vi "Write Scan Configuration.vi"(8 "error in (no error)":errorcluster, 10 "Configuration":T1={"Start"=-0.001, "End"=0.001, "Step"=0.0001, "Delta"=0.0001, "Scan shape"=enum."Sawtooth", "Append measurements"=[]} {"Delta" format="%#_6p"; "Step" format="%#_6p"; "End" format="%#_6p"; "Start" format="%#_6p"}, 11 "Keithley 622x2182 Driver in":refnum<class "Keithley 622x2182 Driver.lvclass">) -> (0 "error out":errorcluster, 3 "Keithley 622x2182 Driver out":refnum<class "Keithley 622x2182 Driver.lvclass">)   [LabVIEW 2021, in "Keithley 622x2182 Driver.lvclass"]
uses:
  Keithley 622x2182 Driver.lvclass
  C:/Git/NHMFL_Core/Libraries/Instruments/Instrument Driver/Instrument Driver.lvclass
  Controls/Stepper Config.ctl
  Keithley 622x2182 Driver.lvclass/Keithley 622x2182 Driver.ctl
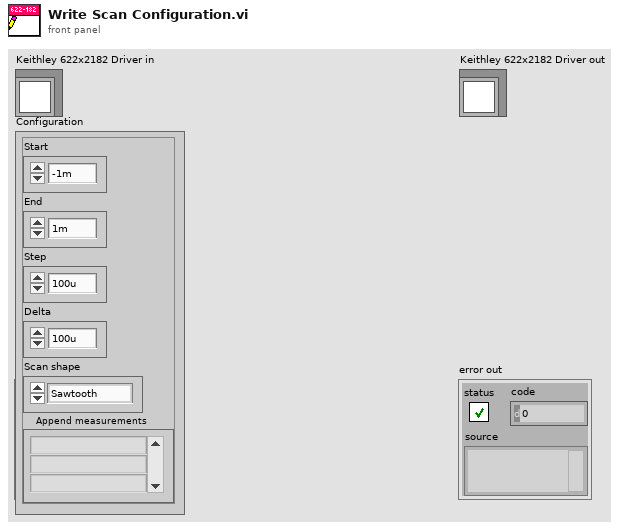
[diagram p1: front panel]
types:
  T1 = typedef "Stepper Config.ctl" = cluster{"Start":dbl, "End":dbl, "Step":dbl, "Delta":dbl, "Scan shape":enum16{"Sawtooth", "Triangular"}, "Append measurements":string[]}
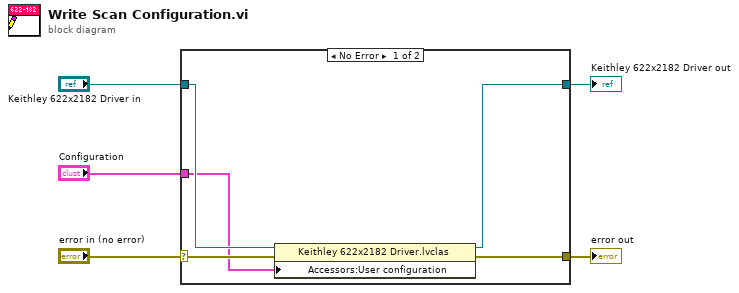
[diagram p0: block diagram]
diagram:
  n1 = case shown="No Error" "error in (no error)" {
    selector: "error in (no error)" -> [w10 w11]
    tunnel: [w9 w11] -> w4
    tunnel: [w7 w12] -> w2
    tunnel: "Keithley 622x2182 Driver in" -> [w8 w12]
    tunnel: "Configuration" -> [w6 _]
    frame No Error {
      n2 = property class="Keithley 622x2182 Driver.lvclas"(reference=w8, error in=w10, "Accessors:User configuration"=w6) -> (reference out=w7:refnum<class "Keithley 622x2182 Driver.lvclass">, error out=w9:errorcluster)
    }
    frame Error {
    }
  }
  "error out" <- w4
  "Keithley 622x2182 Driver out" <- w2
